vi "Test.vi"(10 "Suchstring":string, 11 "String":string) -> (3 "Anzahl der Ersetzungen":i32)   [LabVIEW 2015, in "SysLog.lvlib"]
uses:
  SysLog.lvlib
panel:
  out "Numerisch":i32
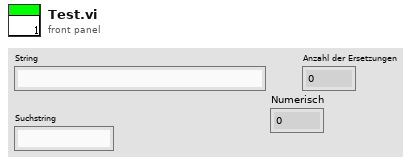
[diagram p1: front panel]
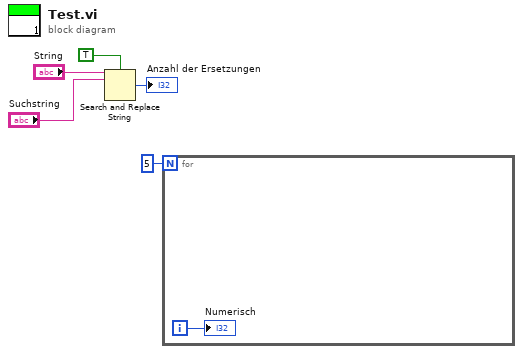
[diagram p0: block diagram]
diagram:
  n1 = Search and Replace String(case sensitive?=TRUE ("Schreibweise ignorieren (F)"), input string="String", search string="Suchstring") -> (number of replacements=→"Anzahl der Ersetzungen":i32)  [unwired: 5 in, 3 out]
  n2 = for {
    N: 5 -> [_]
    i -> [w6]
    "Numerisch" <- w6
  }
